vi "Picture Size Write.vi"(4 "error in (no error)":errorcluster, 5 "Value":T1, 6 "Container State":T3, 7 "Display State In":T2) -> (0 "error out":errorcluster, 3 "Display State Out":T2)   [LabVIEW 2013]
uses:
  <vilib>/_xctls/Container State.ctl
  PicList_State.ctl
  <vilib>/Utility/miscctls.llb/LVBoundsTypeDef.ctl
  PicList.xctl
  <vilib>/_xctls/XControlSupport.lvlib
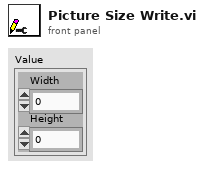
[diagram p1: front panel]
types:
  T1 = typedef "LVBoundsTypeDef.ctl" = cluster{"Width":u32, "Height":u32}
  T2 = typedef "PicList.xctl/PicList_State.ctl" = cluster{"Persistent":cluster{"Pictures":picture[], "Selection":i32, "Selection Layer":picture, "Highlight":i32, "Hover Layer":picture}, "Selection Color":u32, "Highlight Color":u32, "Draw Area Size":T1, "List Ref":refnum<vi>, "Visible":u8}
  T3 = typedef "XControlSupport.lvlib/Container State.ctl" = cluster{"Indicator?":bool, "Run Mode?":bool, " Refnum":refnum<vi>}
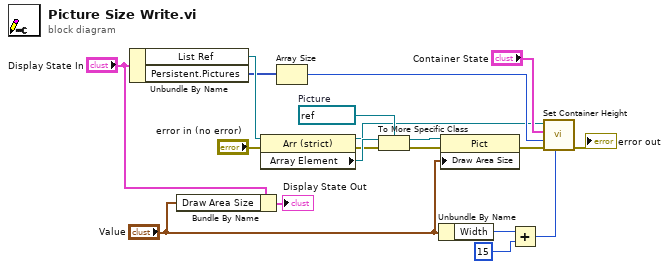
[diagram p0: block diagram]
diagram:
  w15 = refnum<vi> refnum  # Picture
  n1 = Unbundle By Name("Display State In") -> ("List Ref"=w18:refnum<vi>, "Persistent.Pictures"=w6:picture[])
  n2 = Bundle By Name(cluster="Display State In", "Draw Area Size"="Value") -> (→"Display State Out":T2)
  n3 = property class="Arr (strict)"(reference=w18, error in="error in (no error)") -> (reference out=w4:refnum<vi>, error out=w16:errorcluster, "Array Element"=w17:refnum<vi>)
  n4 = Array Size(array=w6) -> (size(s)=w5:i32)
  n5 = To More Specific Class(target class=w15, reference=w17, error in=w16) -> (specific class reference=w13:refnum<vi>, error out=w14:errorcluster)
  n6 = Unbundle By Name("Value") -> ("Width"=w9:u32)
  n7 = property class="Pict"(reference=w13, error in=w14, "Draw Area Size"="Value") -> (error out=w3:errorcluster)  [unwired: 1 out]
  n8 = Add(x=w9, y=u32 15) -> (x+y=w7:u32)
  n9 = call "Set Container Height.vi"("Container Width"=w7, "error in (no error)"=w3, "# of Pictures"=w5, "Container State"="Container State", "Array in"=w4) -> ("error out"=→"error out":errorcluster)  [unwired: 5 in, 1 out]
